vi "get_pose.vi"(6 "Magic offset":i16, 8 "Selector":T1, 9 "Input Trace":sgl[][](array[numeric])) -> (1 "Pose":T2)   [LabVIEW 2013]
uses:
  <vilib>/Analysis/Matrix/Datatypes/RealMatrix.ctl
  testing/pose_source.ctl
  testing/probe_point.ctl
  <vilib>/Analysis/Matrix/Numeric/Conversions/Array To Matrix - RA.vi
  utilities/labview/euler_to_rotation.vi
  <vilib>/Analysis/Matrix/NI_Matrix.lvlib
panel:
  # "Extract one of the  4x4 pose matrices from a trace data record, given  a selection code  (default output pose = 0)"
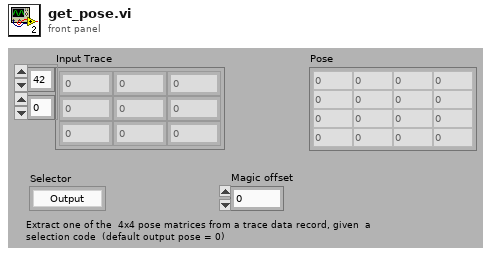
[diagram p1: front panel]
types:
  T1 = typedef "pose_source.ctl" = enum16{"Output", "Handle", "Handle KF", "Goal", "Absolute"}
  T2 = typedef "NI_Matrix.lvlib/RealMatrix.ctl" = dbl[][]
  T3 = typedef "probe_point.ctl" = enum16{"Position (tip)", "Position (RCM)", "Null pos (tip)", "Null pos (RCM)", "V limiter (tip)", "V Limiter (RCM)", "Goal (tip)", "Goal (RCM)", "Link pos 0", "Link pos 1", "KF link pos 0", "KF link pos 1", "Link rate 0", "Link rate 1", "Link residue 0", "Link residue 1", "Link goal 0", "Link goal 1", "Rate limit 0", "Rate limit 1", "Link error 0", "Link error 1", "Controller 0", "Controller 1", "Output 0", "Output 1", "Drive 0", "Drive 1", "Stimulus 0", "Stimulus 1", "Trace data 0", "Trace data 1", "Analog data 0", "Analog data 1", "Status flags", "Light 0", "Light 1", "Light 2", "Light 3", "Light 4", "Light 5", "Goal origin", "Goal rotation 0", "Goal rotation 1", "Goal rotation 2", "Output origin", "Output rotation 0", "Output rotation 1", "Output rotation 2", "Handle origin", "Handle rotation 0", "Handle rotation 1", "Handle rotation 2", "Handle position", "Handle velocity", "Handle acceleration", "Handle angles", "Handle angle rates", "Handle pos residue", "Handle angle residue", "Trace length"}
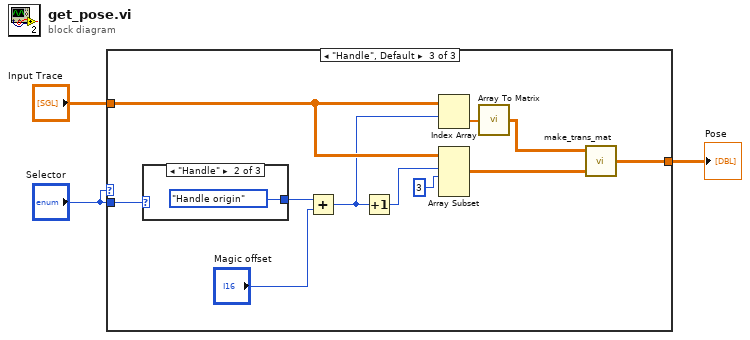
[diagram p0: block diagram]
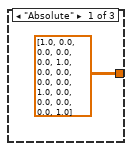
[diagram p2: hidden frame]
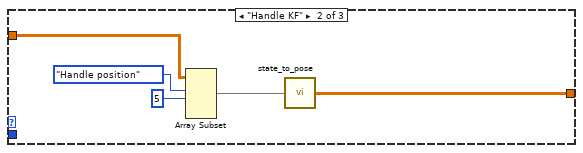
[diagram p3: hidden frame]
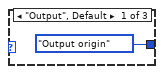
[diagram p4: hidden frame]
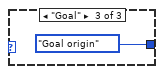
[diagram p5: hidden frame]
diagram:
  n1 = case shown="\"Handle\", Default" "Selector" {
    tunnel: "Input Trace" -> [_ w9 w20]
    tunnel: [T2 [[1.0, 0.0, 0.0, 0.0], [0.0, 1.0, 0.0, 0.0], [0.0, 0.0, 1.0, 0.0], [0.0, 0.0, 0.0, 1.0]] ("Special Matrix") w5 w19] -> w2
    tunnel: "Selector" -> [_ _ w13]
    frame "Absolute" {
    }
    frame "Handle KF" {
      n2 = Array Subset(array=w9, index (row)=probe_point."Handle position" ("Origin index"), length (row)=5 ("length")) -> (w6:sgl[][])  [unwired: 2 in]
      n3 = call "state_to_pose.vi"("Handle State"=w6) -> ("Pose"=w5:T2)
    }
    frame "Handle", Default {
      n4 = case shown="\"Handle\"" w13 {
        tunnel: [probe_point."Output origin" ("Origin index") probe_point."Handle origin" ("Origin index") probe_point."Goal origin" ("Origin index")] -> w12
        frame "Output", Default {
        }
        frame "Handle" {
        }
        frame "Goal" {
        }
      }
      n5 = Add(x=w12, y="Magic offset") -> (x+y=w10:u16)
      n6 = Increment(x=w10) -> (x+1=w14:u16)
      n7 = Index Array(array=w20, index (row)=w10) -> (element=w16:sgl[])  [unwired: 1 in]
      n8 = Array Subset(array=w20, index (row)=w14, length (row)=3 ("length")) -> (w17:sgl[][])  [unwired: 2 in]
      n9 = call-poly <vilib>:"Array To Matrix.vi"("Real 1D Array"=w16) -> ("Real Matrix (Column Vector)"=w15:T2)
      n10 = call "make_trans_mat.vi"("Rotation"=w17, "Translation"=w15) -> ("Transform"=w19:T2)  [unwired: 3 out]
    }
  }
  "Pose" <- w2
